vi "client.vi"() -> ()   [LabVIEW 2018]
uses:
  <vilib>/httpClient/LabVIEWHTTPClient.lvlib
panel:
  out "Waveform Graph":dbl[](graph)
  out "Array":dbl[][](array[numeric])
  out "body":string
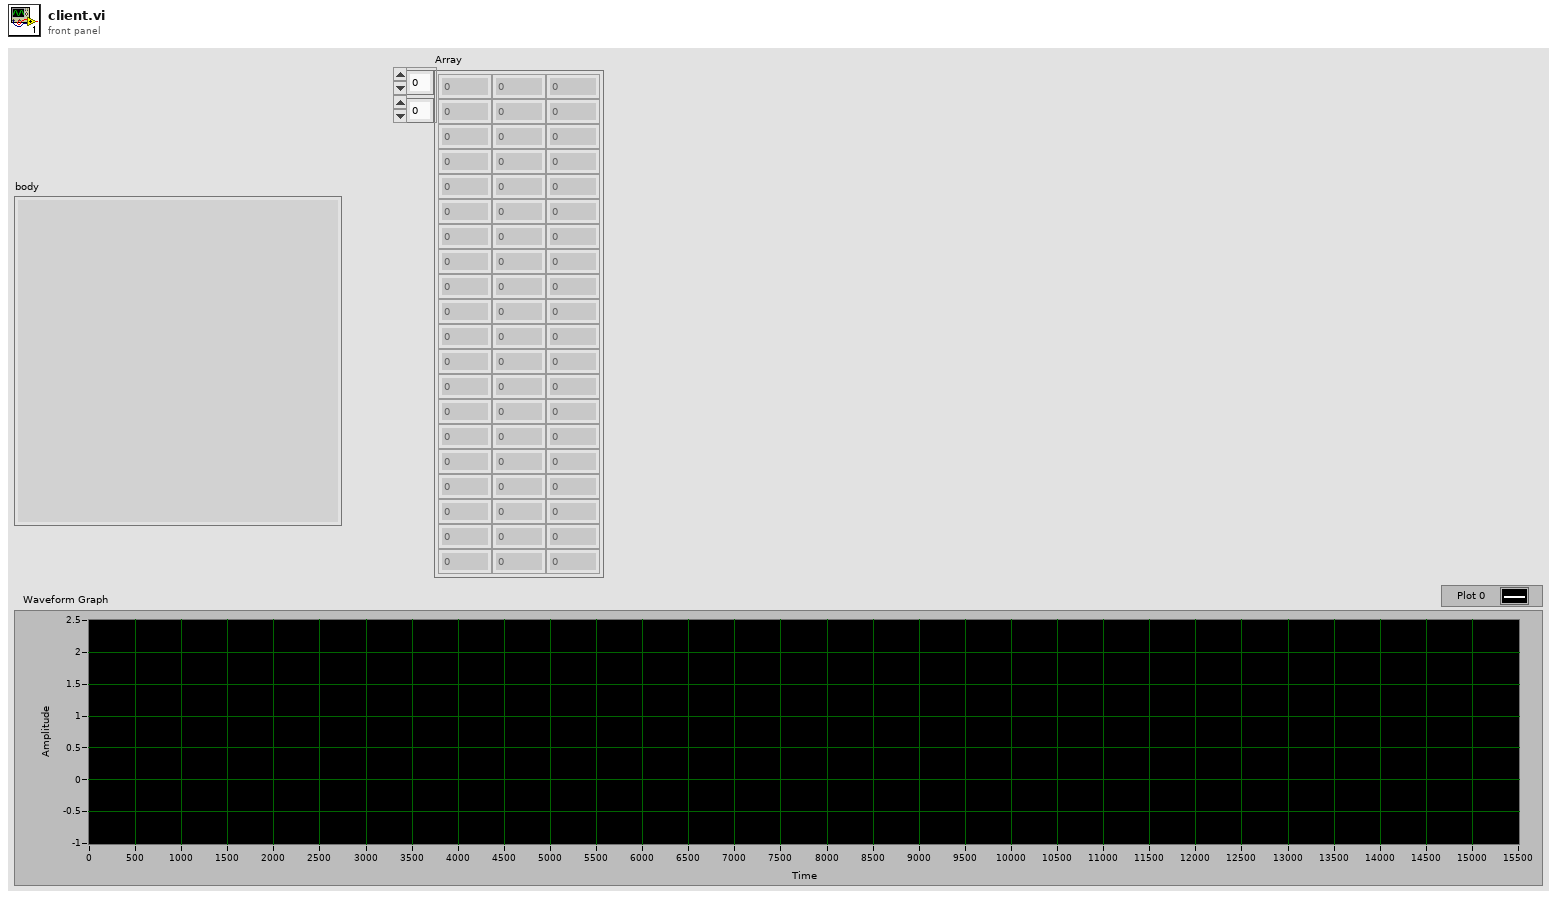
[diagram p1: front panel]
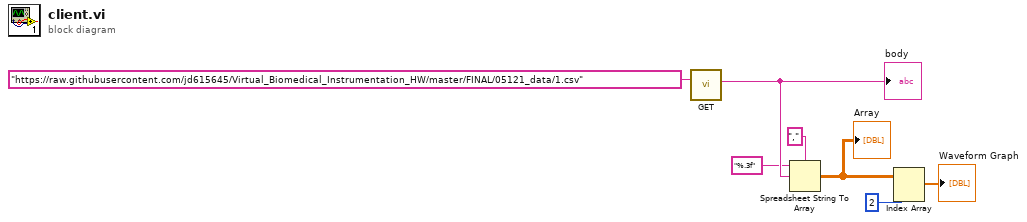
[diagram p0: block diagram]
diagram:
  n1 = call <vilib>:"GET.vi"("url"="https://raw.githubusercontent.com/jd615645/Virtual_Biomedical_Instrumentation_HW/master/FINAL/05121_data/1.csv") -> ("body"=w6:string)  [unwired: 11 in, 3 out]
  "body" <- w6
  n2 = Spreadsheet String To Array(delimiter (Tab)=",", format string="%.3f", spreadsheet string=w6) -> (array=w1:dbl[][])  [unwired: 1 in]
  "Array" <- w1
  n3 = Index Array(array=w1, index (col)=2) -> (element=→"Waveform Graph":dbl[])  [unwired: 1 in]
